vi "Read data.vi"(8 "error in (no error)":errorcluster, 11 "Node in":refnum<class "DoublyNode.lvclass">) -> (0 "error out":errorcluster, 2 "data":dbl, 3 "Node out":refnum<class "DoublyNode.lvclass">)   [LabVIEW 2021, in "DoublyNode.lvclass"]
uses:
  DoublyNode.lvclass
  DoublyNode.lvclass/DoublyNode.ctl
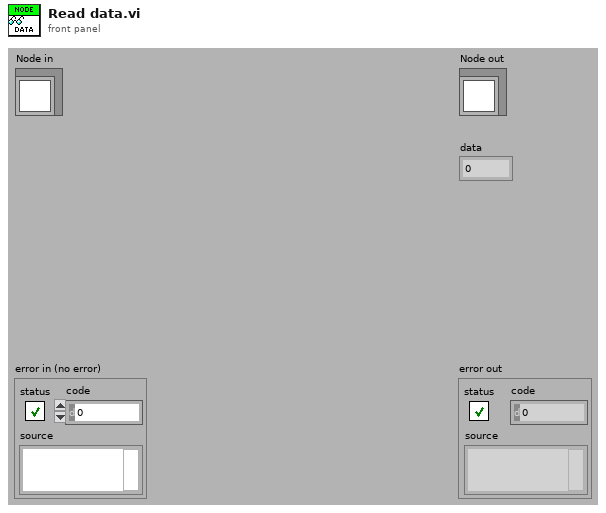
[diagram p1: front panel]
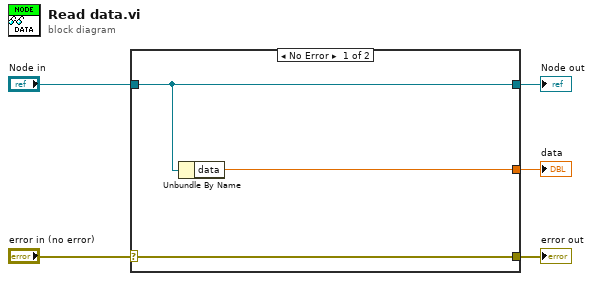
[diagram p0: block diagram]
diagram:
  n1 = case shown="No Error" "error in (no error)" {
    selector: "error in (no error)" -> [w8 w9]
    tunnel: [w8 w9] -> w4
    tunnel: [w7 w10] -> w2
    tunnel: "Node in" -> [w7 w10]
    tunnel: [w6 _] -> w1
    frame No Error {
      n2 = Unbundle By Name(w7) -> ("data"=w6:dbl)
    }
    frame Error {
    }
  }
  "error out" <- w4
  "Node out" <- w2
  "data" <- w1
